vi "Read Joystick.vi"(8 "Joystick Deadbanded Value (default of 0.1)":dbl, 11 "Joystick L 1 DevRef":T1) -> (1 "Joystick L 2 X Axis":dbl, 2 "Joystick L 1 Y Axis":dbl, 3 "Joystick L 1 X Axis":dbl)   [LabVIEW 2014]
uses:
  <vilib>/Rock Robotics/WPI/Joystick/WPI_JoystickDevRef.ctl
  <vilib>/Rock Robotics/WPI/Joystick/WPI_JoystickDeviceEnum.ctl
  Global Variables.vi
  <vilib>/Rock Robotics/WPI/Joystick/WPI_JoystickGetSetRefNum.vi
  <vilib>/Utility/file.llb/Write To Spreadsheet File (DBL).vi
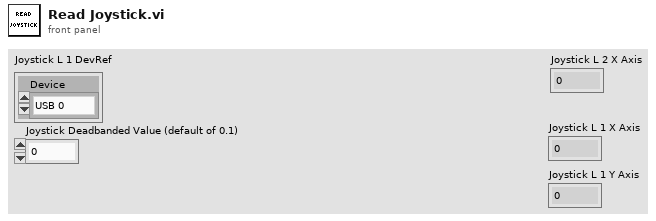
[diagram p1: front panel]
types:
  T1 = typedef "WPI_JoystickDevRef.ctl" = cluster{"Device":T2}
  T2 = typedef "WPI_JoystickDeviceEnum.ctl" = enum16{"USB 0", "USB 1", "USB 2", "USB 3", "USB 4", "USB 5"}
  T3 = cluster{"Buttons[0]":bool, "Buttons[1]":bool, "Buttons[2]":bool, "Buttons[3]":bool, "Buttons[4]":bool, "Buttons[5]":bool, "Buttons[6]":bool, "Buttons[7]":bool, "Buttons[8]":bool}
  T4 = cluster{"Axes[0]":dbl, "Axes[1]":dbl, "Axes[2]":dbl, "Axes[3]":dbl, "Axes[4]":dbl, "Axes[5]":dbl, "Axes[6]":dbl, "Axes[7]":dbl, "Axes[8]":dbl}
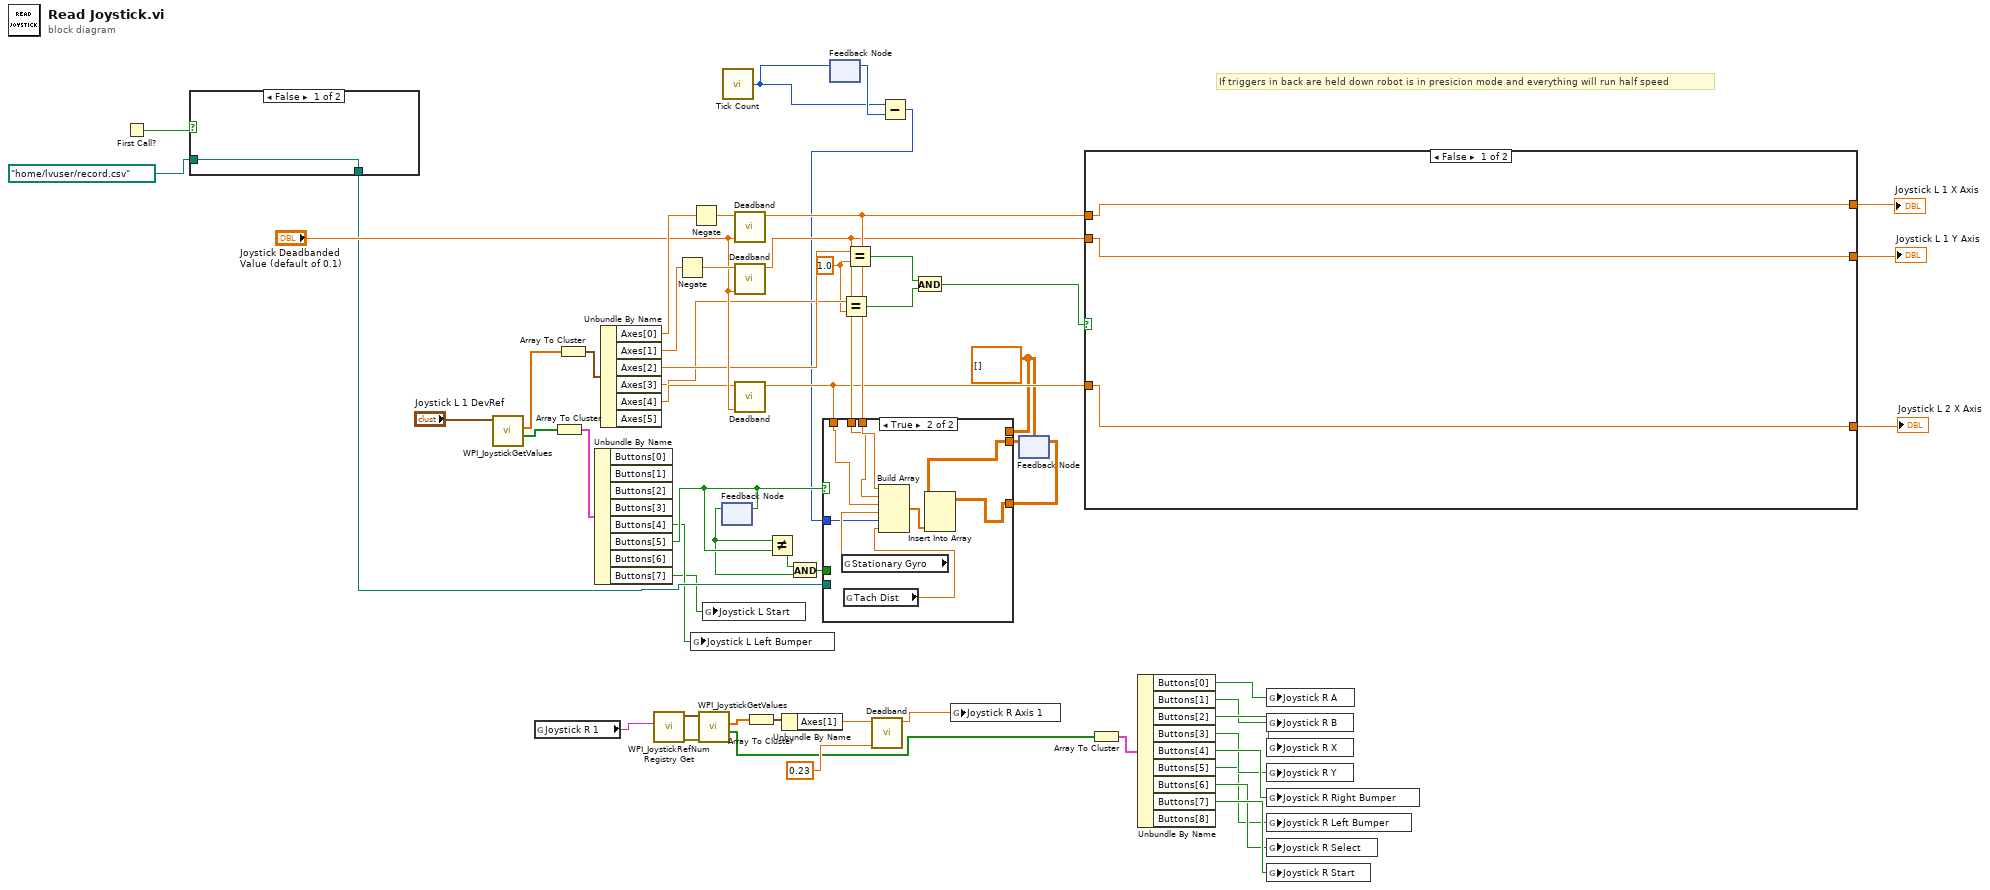
[diagram p0: block diagram]
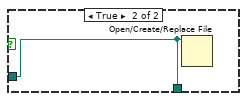
[diagram p2: hidden frame]
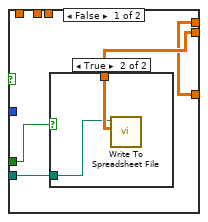
[diagram p3: hidden frame]
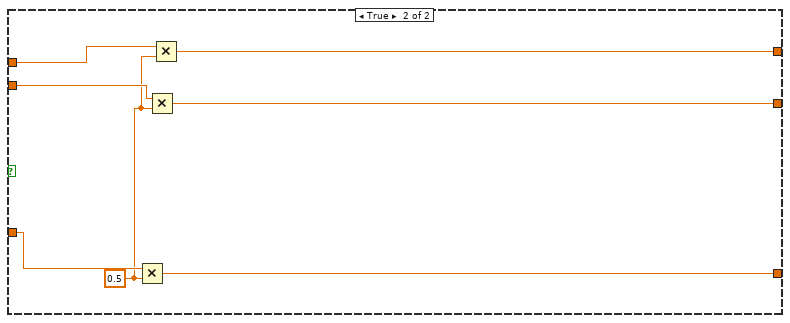
[diagram p5: hidden frame]
diagram:
  w4 = dbl[][] []
  w26 = 1.0 ("y")
  # "If triggers in back are held down robot is in presicion mode and everything will run half speed"
  n1 = First Call?() -> (First Call?: T/F=w10:bool)
  n2 = case shown="False" w10 {
    tunnel: [w57 w58] -> w9
    tunnel: path "/home/lvuser/record.csv" ("file path (use dialog)") -> [w57 w58]
    frame False {
    }
    frame True {
      n3 = Open/Create/Replace File(file path (use dialog)=w58) -> ()  [unwired: 5 in, 3 out]
    }
  }
  n4 = call <vilib>:"WPI_JoystickGetValues.vi"("JoystickDevRef"="Joystick L 1 DevRef") -> ("Buttons"=w53:bool[], "Axes"=w55:dbl[])  [unwired: 6 in, 3 out]
  n5 = global read "Global Variables.vi" "Joystick R 1"() -> (w44:string)
  n6 = Array To Cluster(array=w53) -> (cluster=w52:T3)
  n7 = Array To Cluster(array=w55) -> (cluster=w54:T4)
  n8 = Unbundle By Name(w52) -> ("Buttons[4]"=w6:bool, "Buttons[5]"=w13:bool, "Buttons[7]"=w5:bool)  [unwired: 5 out]
  n9 = Unbundle By Name(w54) -> ("Axes[0]"=w51:dbl, "Axes[1]"=w48:dbl, "Axes[2]"=w28:dbl, "Axes[3]"=w27:dbl, "Axes[4]"=w29:dbl)  [unwired: 1 out]
  n10 = call <vilib>:"WPI_JoystickRefNum Registry Get.vi"("refnum name"=w44) -> ("error out"=w43:errorcluster, "JoystickDevRef"=w42:T1)  [unwired: 9 in]
  n11 = Negate(x=w48) -> (-x=w49:dbl)
  n12 = Negate(x=w51) -> (-x=w50:dbl)
  n13 = global write "Global Variables.vi" "Joystick L Left Bumper"(w6) -> ()
  n14 = call <vilib>:"WPI_JoystickGetValues.vi"("error in (no error)"=w43, "JoystickDevRef"=w42) -> ("Buttons"=w31:bool[], "Axes"=w45:dbl[])  [unwired: 5 in, 3 out]
  n15 = global write "Global Variables.vi" "Joystick L Start"(w5) -> ()
  n16 = feedback #1() -> (w12:bool)  [unwired: 1 in]
  n17 = feedback-in #1(w13) -> ()
  n18 = call "Tick Count"() -> ("Tick Count(mSec)"=w2:u32)
  n19 = call "Deadband.vi"("Value to Deadband (default of 0.1)"="Joystick Deadbanded Value (default of 0.1)", "Value"=w50) -> ("Deadbanded Value"=w19:dbl)  [unwired: 9 in]
  n20 = call "Deadband.vi"("Value to Deadband (default of 0.1)"="Joystick Deadbanded Value (default of 0.1)", "Value"=w49) -> ("Deadbanded Value"=w16:dbl)  [unwired: 9 in]
  n21 = call "Deadband.vi"("Value to Deadband (default of 0.1)"="Joystick Deadbanded Value (default of 0.1)", "Value"=w29) -> ("Deadbanded Value"=w15:dbl)  [unwired: 9 in]
  n22 = Array To Cluster(array=w45) -> (cluster=w46:T4)
  n23 = Not Equal?(x=w12, y=w13) -> (x != y?=w14:bool)
  n24 = Unbundle By Name(w46) -> ("Axes[1]"=w40:dbl)
  n25 = And(x=w14, y=w12) -> (x .and. y?=w11:bool)
  n26 = feedback-in #2(w2) -> ()
  n27 = feedback #2() -> (w3:u32)  [unwired: 1 in]
  n28 = Equal?(x=w27, y=w26) -> (x = y?=w24:bool)
  n29 = Equal?(x=w28, y=w26) -> (x = y?=w25:bool)
  n30 = call "Deadband.vi"("Value to Deadband (default of 0.1)"=0.23, "Value"=w40) -> ("Deadbanded Value"=w39:dbl)  [unwired: 9 in]
  n31 = Subtract(x=w2, y=w3) -> (x-y=w1:u32)
  n32 = And(x=w25, y=w24) -> (x .and. y?=w23:bool)
  n33 = global write "Global Variables.vi" "Joystick R Axis 1"(w39) -> ()
  n34 = feedback #3(w4) -> (w17:dbl[][])
  n35 = case shown="True" w13 {
    tunnel: w19 -> [_ w71]
    tunnel: [w59 w73] -> w18
    tunnel: w17 -> [w61 w72]
    tunnel: w16 -> [_ w70]
    tunnel: w15 -> [_ w69]
    tunnel: w11 -> [w62 _]
    tunnel: w9 -> [w60 _]
    tunnel: w4 -> [w59 _]
    tunnel: w1 -> [_ w66]
    frame False {
      n36 = case shown="True" w62 {
        tunnel: w61 -> [_ w64]
        tunnel: w60 -> [_ w63]
        frame False {
        }
        frame True {
          n37 = call-poly <vilib>:"Write To Spreadsheet File.vi"("2D data"=w64, "file path (dialog if empty)"=w63) -> ()  [unwired: 6 in, 1 out]
        }
      }
    }
    frame True {
      n38 = global read "Global Variables.vi" "Stationary Gyro"() -> (w67:dbl)
      n39 = global read "Global Variables.vi" "Tach Dist"() -> (w65:dbl)
      n40 = Build Array(w71, w70, w69, w67, w66, w65) -> (w68:dbl[])
      n41 = Insert Into Array(array=w72, new element=w68) -> (w73:dbl[][])  [unwired: 2 in]
    }
  }
  n42 = feedback-in #3(w18) -> ()
  n43 = case shown="False" w23 {
    tunnel: w15 -> [w74 w83]
    tunnel: w16 -> [w75 w82]
    tunnel: w19 -> [w76 w80]
    tunnel: [w76 w79] -> w22
    tunnel: [w75 w78] -> w21
    tunnel: [w74 w77] -> w20
    frame False {
    }
    frame True {
      w81 = 0.5 ("y")
      n44 = Multiply(x=w83, y=w81) -> (x*y=w77:dbl)
      n45 = Multiply(x=w82, y=w81) -> (x*y=w78:dbl)
      n46 = Multiply(x=w80, y=w81) -> (x*y=w79:dbl)
    }
  }
  "Joystick L 1 Y Axis" <- w21
  "Joystick L 1 X Axis" <- w22
  "Joystick L 2 X Axis" <- w20
  n47 = Array To Cluster(array=w31) -> (cluster=w32:T3)
  n48 = Unbundle By Name(w32) -> ("Buttons[0]"=w30:bool, "Buttons[1]"=w33:bool, "Buttons[2]"=w34:bool, "Buttons[3]"=w35:bool, "Buttons[4]"=w36:bool, "Buttons[5]"=w7:bool, "Buttons[6]"=w37:bool, "Buttons[7]"=w38:bool)  [unwired: 1 out]
  n49 = global write "Global Variables.vi" "Joystick R A"(w30) -> ()
  n50 = global write "Global Variables.vi" "Joystick R B"(w33) -> ()
  n51 = global write "Global Variables.vi" "Joystick R X"(w34) -> ()
  n52 = global write "Global Variables.vi" "Joystick R Y"(w35) -> ()
  n53 = global write "Global Variables.vi" "Joystick R Right Bumper"(w36) -> ()
  n54 = global write "Global Variables.vi" "Joystick R Left Bumper"(w7) -> ()
  n55 = global write "Global Variables.vi" "Joystick R Select"(w37) -> ()
  n56 = global write "Global Variables.vi" "Joystick R Start"(w38) -> ()
